vi "main.vi"() -> ()   [LabVIEW 2016]
uses:
  <vilib>/Instr/_visa.llb/VISA Configure Serial Port (Instr).vi
panel:
  in  "OK Button":bool
  in  "Numeric":dbl
  in  "pos":dbl[](array[numeric])
  in  "UART PORT":refnum<visa-resource-name>
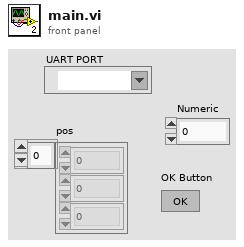
[diagram p1: front panel]
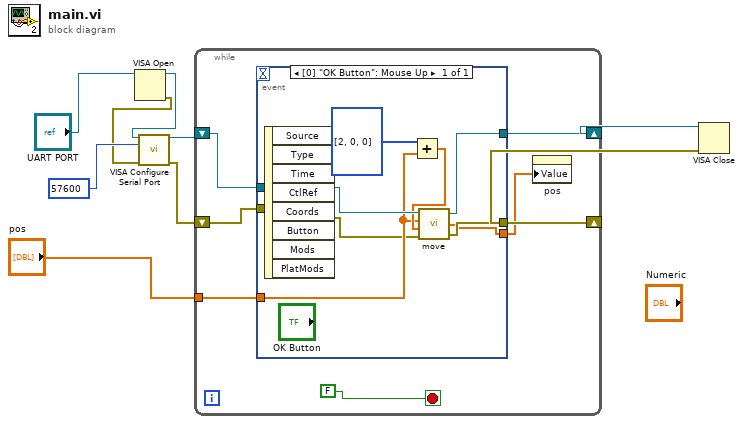
[diagram p0: block diagram]
diagram:
  n1 = VISA Open(VISA resource name="UART PORT") -> (VISA resource name=w6:refnum<visa-resource-name>, error out=w7:errorcluster)  [unwired: 4 in]
  n2 = call-poly "VISA Configure Serial Port"("VISA resource name"=w6, "baud rate (9600)"=57600, "error in (no error)"=w7) -> ("VISA resource name out"=w5:refnum<visa-resource-name>, "error out"=w4:errorcluster)  [unwired: 11 in]
  n3 = while {
    shift-right: [w12] -> w3
    shift-left: w5 -> [w16]
    shift-right: [w11] -> w2
    shift-left: w4 -> [w15]
    tunnel: "pos" -> [w13]
    stop <- FALSE stop-if-true
    n4 = event shown="[0] \"OK Button\": Mouse Up" {
      selector: _ -> [_]
      dyn-events: _ -> [_]
      timeout: _ -> [_]
      tunnel: w16 -> [w24]
      tunnel: w15 -> [w20]
      tunnel: w13 -> [w21]
      tunnel: [w19] -> w12
      tunnel: [w18] -> w11
      tunnel: [w17] -> w10
      event "OK Button": Mouse Up {
        n5 = event-data() -> ()  [unwired: 1 in, 8 out]
        n6 = Add(x=i32[] [2, 0, 0], y=w21) -> (x+y=w22:dbl[])
        n7 = call "move.vi"("error in (no error)"=w20, "P01"=w22, "P0"=w21, "UART PORT in"=w24) -> ("error out"=w18:errorcluster, "P1"=w17:dbl[], "UART PORT out"=w19:refnum<visa-resource-name>)
      }
    }
    n8 = property on="pos" class="Arr (strict)"("Value"=w10) -> ()  [unwired: 2 in, 2 out]
  }
  n9 = VISA Close(VISA resource name=w3, error in (no error)=w2) -> ()  [unwired: 1 out]
